vi "JustTesting.vi"() -> ()   [LabVIEW 2022 SP3]
uses:
  _LVsubs/PythonCtrl.ctl
  _LVsubs/Processors.ctl
panel:
  out "return value 2":string
  out "return value":string[](array[string])
  out "Text read":string
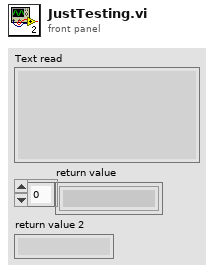
[diagram p1: front panel]
types:
  T1 = typedef "PythonCtrl.ctl" = cluster{"session":refnum<k35>, "PyPath":path, "Processor":T2, "Port":string, "version":string}
  T2 = typedef "Processors.ctl" = enum16{"SPIKE", "Pi", "Pi_ssh", "OpenMV", "Dunio"}
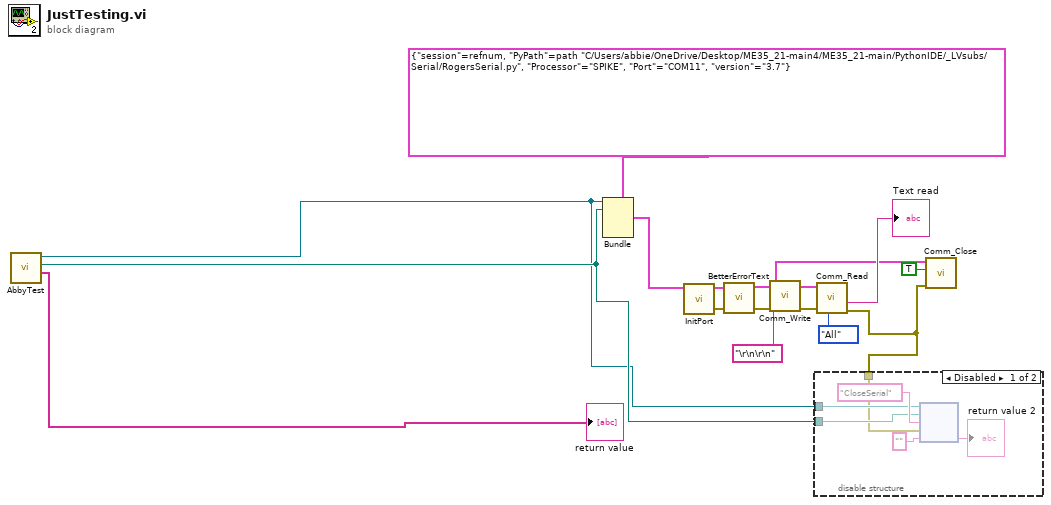
[diagram p0: block diagram]
diagram:
  n1 = call "AbbyTest.vi"() -> ("Array"=→"return value":string[], "appended path"=w5:path, "Refnum out"=w4:refnum<k35>)  [unwired: 9 in]
  n2 = Bundle(cluster=T1 {"session"=refnum, "PyPath"=path "C:/Users/abbie/OneDrive/Desktop/ME35_21-main4/ME35_21-main/PythonIDE/_LVsubs/Serial/RogersSerial.py", "Processor"=enum."SPIKE", "Port"="COM11", "version"="3.7"} ("Python"), "session"=w4, "PyPath"=w5) -> (w7:T1)  [unwired: 3 in]
  n3 = call "InitPort.vi"("Python"=w7) -> ("error out"=w11:errorcluster, "Python out"=w14:T1)  [unwired: 8 in, 1 out]
  n4 = call "BetterErrorText.vi"("error in (no error)"=w11, "Python"=w14) -> ("Python out"=w3:T1)  [unwired: 8 in, 1 out]
  n5 = call "Comm_Write.vi"("error in (no error)"=w11, "Text to write"="\r\n\r\n", "Python"=w3) -> ("error out"=w10:errorcluster)  [unwired: 7 in, 1 out]
  n6 = call "Comm_Read.vi"("Task"=enum16{"Instant", "All", "AllFast", "Params"}."All", "error in (no error)"=w10, "Python"=w3) -> ("error out"=w2:errorcluster, "Text read"=→"Text read":string)  [unwired: 7 in]
  n7 = disable-structure shown="Disabled" {
    disable-tunnel: w5 -> [w18 _]
    disable-tunnel: w4 -> [w17 _]
    disable-tunnel: w2 -> [w15 _]
    frame Disabled {
      n8 = node(w17, w18, "CloseSerial" ("function name"), w15, "" ("function name")) -> (→"return value 2":string)  [unwired: 4 out]
    }
    frame Enabled {
    }
  }
  n9 = call "Comm_Close.vi"("error in (no error)"=w2, "Show Err?"=TRUE, "Python in"=w3) -> ()  [unwired: 7 in, 2 out]
